vi "Write right in tunnels.vi"(5 "right in tunnels":refnum<class "FlatSequenceInnerTunnel.lvclass">[](array[class]), 9 "FlatSequenceFrame in":refnum<class "FlatSequenceFrame.lvclass">) -> (3 "FlatSequenceFrame out":refnum<class "FlatSequenceFrame.lvclass">)   [LabVIEW 2014, in "FlatSequenceFrame.lvclass"]
uses:
  FlatSequenceFrame.lvclass
  FlatSequenceInnerTunnel/FlatSequenceInnerTunnel.lvclass
  FlatSequenceFrame.lvclass/FlatSequenceFrame.ctl
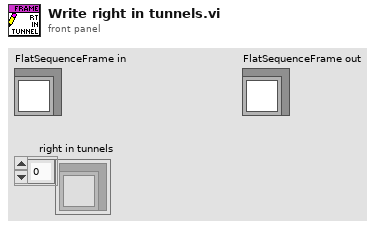
[diagram p1: front panel]
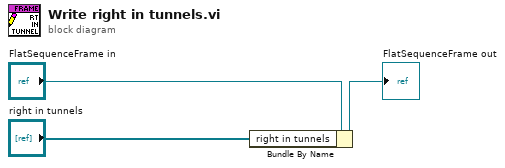
[diagram p0: block diagram]
diagram:
  n1 = Bundle By Name(cluster="FlatSequenceFrame in", "right in tunnels"="right in tunnels") -> (→"FlatSequenceFrame out":refnum<class "FlatSequenceFrame.lvclass">)
